vi "Main Reversi.vi"(6 "Highlight Possible Moves?":bool, 8 "error in (no error)":errorcluster, 9 "Wait per Turn (ms)":u32(slide) scale=0.0..1000.0, 10 "Games Per Match":u32=1 min=1 max=1000, 11 "Game Mode":T1(ring)) -> (0 "error out":errorcluster)   [LabVIEW 2020, in "Reversi.lvlib" / "Reversi.lvclass"]
uses:
  Reversi.lvclass
  Space Ring.ctl
  Reversi.lvclass/Reversi.ctl
  <vilib>/Utility/miscctls.llb/LVMapReplaceAction.ctl
  Player/Player.lvclass
panel:
  in  "Close":bool
  out "Win Count":i32(listbox)
  out "Running Stats":i32(listbox)
  out "Current Turn":T2
  in  "Stop":bool
  out "Board":T2[][](array[typedef])
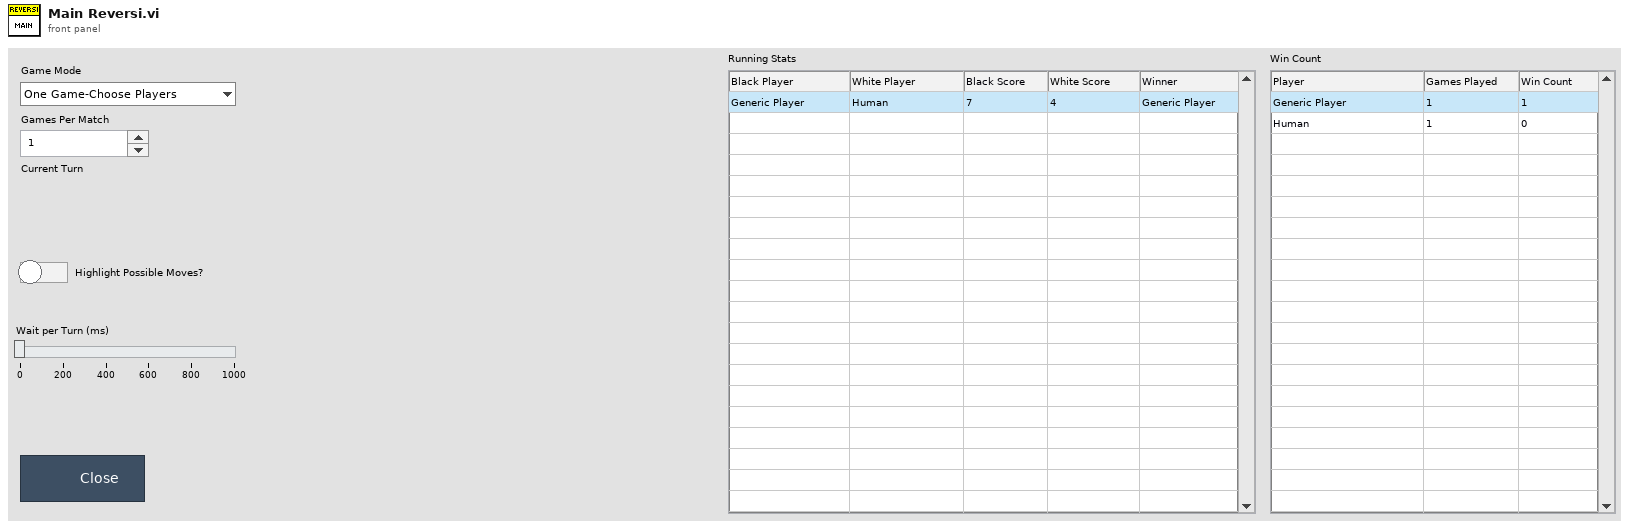
[diagram p1: front panel]
types:
  T1 = enum16{"One Game-Choose Players", "Challenge Matches (All Players)"}
  T2 = typedef "Reversi.lvlib/Reversi.lvclass/Space Ring.ctl" = u16
  T3 = cluster{"Black":refnum<class "Player.lvclass">, "White":refnum<class "Player.lvclass">}
  T4 = cluster{"Black":refnum<class "Player.lvclass">, "White":refnum<class "Player.lvclass">}[]
  T5 = cluster{"Player out":refnum<class "Player.lvclass">, "Player out":refnum<class "Player.lvclass">}
  T6 = typedef "LVMapReplaceAction.ctl" = enum32{"Modify Entry only if found", "Add or Modify Entry", "Delete Entry"}
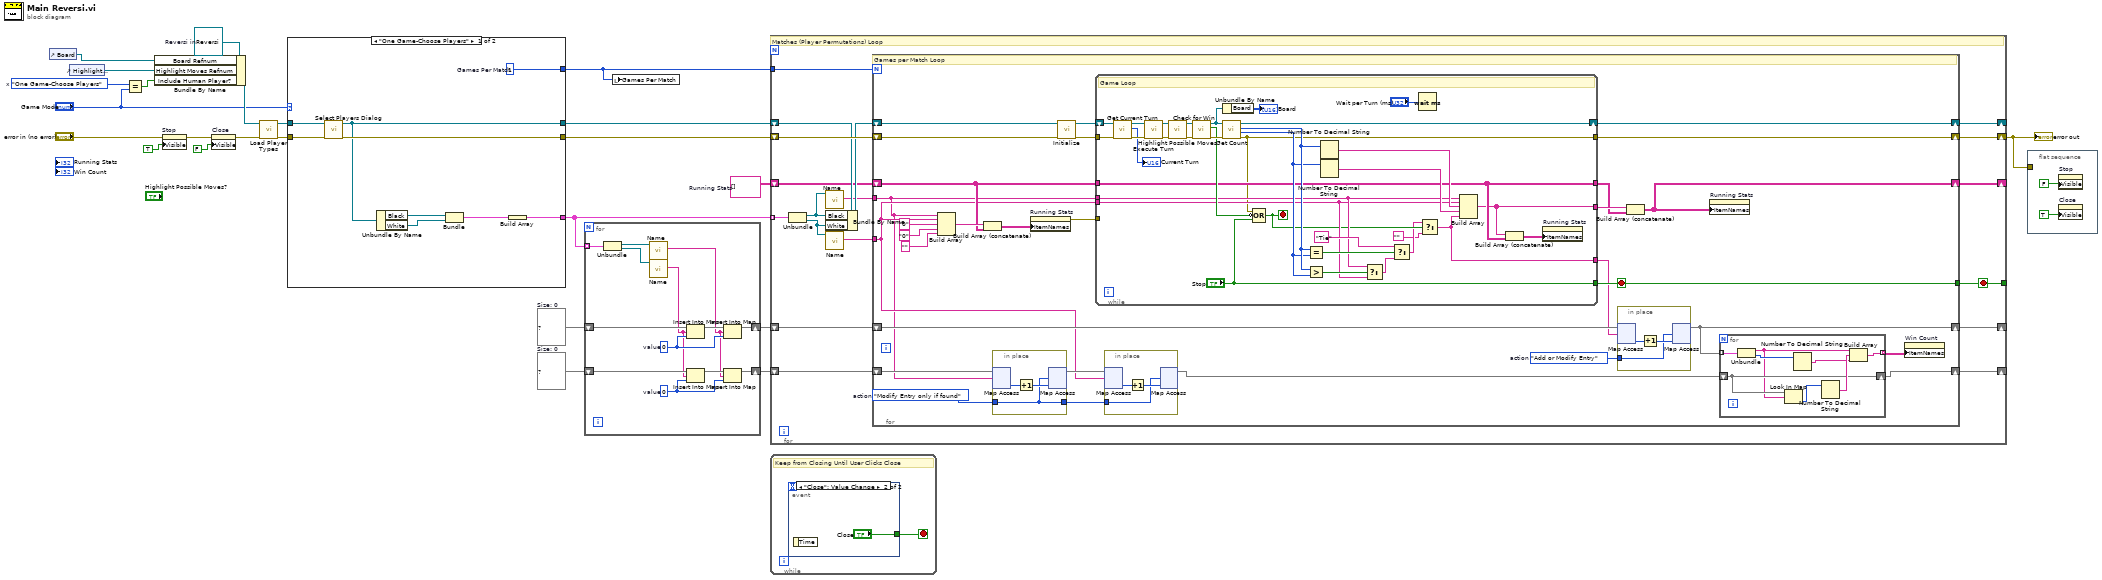
[diagram p0: block diagram]
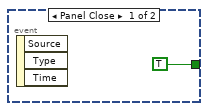
[diagram p2: hidden frame]
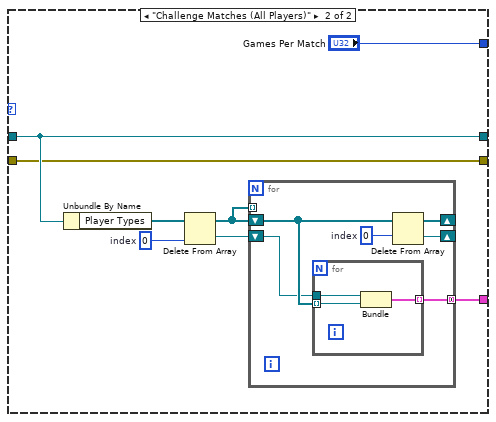
[diagram p3: hidden frame]
diagram:
  w24 = refnum<class "Reversi.lvclass"> refnum  # Reversi in
  w11 = T1."One Game-Choose Players"  # x
  w14 = map{string, i32} {}  # Size: 0
  w17 = map{string, i32} {}  # Size: 0
  w18 = string[][] []  # Running Stats
  n1 = control-ref of="Board"() -> (w6:refnum<vi>)
  n2 = control-ref of="Highlight Possible Moves?"() -> (w5:refnum<vi>)
  n3 = Equal?(x=w11, y="Game Mode") -> (x = y?=w10:bool)
  n4 = Bundle By Name(cluster=w24, "Board Refnum"=w6, "Highlight Moves Refnum"=w5, "Include Human Player?"=w10) -> (w23:refnum<class "Reversi.lvclass">)
  n5 = property on="Stop" class="Bool"(error in="error in (no error)", "Visible"=TRUE) -> (error out=w3:errorcluster)  [unwired: 1 in, 1 out]
  n6 = property on="Close" class="Bool"(error in=w3, "Visible"=FALSE) -> (error out=w4:errorcluster)  [unwired: 1 in, 1 out]
  n7 = call "Load Player Types.vi"("error in"=w4, "Reversi in"=w23) -> ("error out"=w21:errorcluster, "Reversi out"=w22:refnum<class "Reversi.lvclass">)  [unwired: 8 in]
  n8 = case shown="\"One Game-Choose Players\"" "Game Mode" {
    tunnel: [w26 w41] -> w16
    tunnel: w22 -> [w33 w36]
    tunnel: w21 -> [w32 w35]
    tunnel: [w30 w36] -> w20
    tunnel: [w31 w35] -> w19
    tunnel: [w25 "Games Per Match"] -> w9
    frame "One Game-Choose Players" {
      w25 = u32 1  # Games Per Match
      n9 = call "Select Players Dialog.vi"("error in (no error)"=w32, "Reversi in"=w33) -> ("error out"=w31:errorcluster, "Reversi out"=w30:refnum<class "Reversi.lvclass">)  [unwired: 8 in]
      n10 = Unbundle By Name(w30) -> ("Black"=w29:refnum<class "Player.lvclass">, "White"=w28:refnum<class "Player.lvclass">)
      n11 = Bundle("Black"=w29, "White"=w28) -> (w27:T3)  [unwired: 1 in]
      n12 = Build Array(w27) -> (w26:T4)
    }
    frame "Challenge Matches (All Players)" {
      w39 = 0  # index
      n13 = Unbundle By Name(w36) -> ("Player Types"=w40:refnum<class "Player.lvclass">[])
      n14 = Delete From Array(array=w40, index=w39) -> (deleted portion=w38:refnum<class "Player.lvclass">, array with subset deleted=w37:refnum<class "Player.lvclass">[])  [unwired: 1 in]
      n15 = for {
        shift-right: [w45] -> _
        shift-left: w37 -> [w46]
        tunnel: [w47] -> w41 mode=concatenating
        shift-right: [w42] -> _
        shift-left: w38 -> [w44]
        tunnel: w37 -> [_] mode=indexing
        w43 = 0  # index
        n16 = for {
          tunnel: w44 -> [w50]
          tunnel: w46 -> [w49] mode=indexing
          tunnel: [w48] -> w47 mode=indexing
          n17 = Bundle("Player out"=w50, "Player out"=w49) -> (w48:T5)  [unwired: 1 in]
        }
        n18 = Delete From Array(array=w46, index=w43) -> (deleted portion=w42:refnum<class "Player.lvclass">, array with subset deleted=w45:refnum<class "Player.lvclass">[])  [unwired: 1 in]
      }
    }
  }
  n19 = for {
    tunnel: w16 -> [w63] mode=indexing
    shift-right: [w57] -> w15
    shift-left: w17 -> [w60]
    shift-right: [w53] -> w13
    shift-left: w14 -> [w54]
    w56 = 0  # value
    w58 = 0  # value
    n20 = Unbundle(w63) -> ("Player out"=w62:refnum<class "Player.lvclass">, "Player out"=w61:refnum<class "Player.lvclass">)
    n21 = call-dynamic "Name.vi"("Player in"=w62) -> ("Name"=w52:string)  [unwired: 8 in, 2 out]
    n22 = call-dynamic "Name.vi"("Player in"=w61) -> ("Name"=w51:string)  [unwired: 8 in, 2 out]
    n23 = Insert Into Map(map in=w60, key=w51, value=w58) -> (map out=w59:map{string, i32})  [unwired: 2 out]
    n24 = Insert Into Map(map in=w54, key=w51, value=w56) -> (map out=w55:map{string, i32})  [unwired: 2 out]
    n25 = Insert Into Map(map in=w59, key=w52, value=w58) -> (map out=w57:map{string, i32})  [unwired: 2 out]
    n26 = Insert Into Map(map in=w55, key=w52, value=w56) -> (map out=w53:map{string, i32})  [unwired: 2 out]
  }
  n27 = local write "Games Per Match"(w9) -> ()
  n28 = for {
    shift-right: [w81] -> w1
    shift-left: w19 -> [w79]
    shift-right: [w80] -> _
    shift-left: w20 -> [w76]
    tunnel: w16 -> [w77] mode=indexing
    tunnel: w9 -> [w78]
    shift-right: [w69] -> _
    shift-left: w18 -> [w70]
    shift-right: [w67] -> _
    shift-left: w15 -> [w68]
    shift-right: [w65] -> _
    shift-left: w13 -> [w66]
    tunnel: [w64] -> _
    stop <- w64 stop-if-true
    # "Matches (Player Permutations) Loop"
    n29 = Unbundle(w77) -> ("Player out"=w74:refnum<class "Player.lvclass">, "Player out"=w73:refnum<class "Player.lvclass">)
    n30 = call-dynamic "Name.vi"("Player in"=w74) -> ("Name"=w72:string)  [unwired: 8 in, 2 out]
    n31 = Bundle By Name(cluster=w76, "Black"=w74, "White"=w73) -> (w75:refnum<class "Reversi.lvclass">)
    n32 = call-dynamic "Name.vi"("Player in"=w73) -> ("Name"=w71:string)  [unwired: 8 in, 2 out]
    n33 = for {
      N: w78 -> [_]
      tunnel: [w105] -> w64
      shift-right: [w110] -> w80
      shift-left: w75 -> [w109]
      shift-right: [w111] -> w81
      shift-left: w79 -> [w107]
      tunnel: w72 -> [w82]
      tunnel: w71 -> [w85]
      shift-right: [w96] -> w69
      shift-left: w70 -> [w100]
      shift-right: [w91] -> w67
      shift-left: w68 -> [w94]
      shift-right: [w83] -> w65
      shift-left: w66 -> [w89]
      stop <- w105 stop-if-true
      w88 = LVMapReplaceAction."Modify Entry only if found"  # action
      w92 = LVMapReplaceAction."Add or Modify Entry"  # action
      # "Games per Match Loop"
      n34 = Build Array(w82, w85, "0", "0", "") -> (w101:string[])
      n35 = Build Array (concatenate)(w101, w100) -> (w99:string[][])
      n36 = in-place {
        in-place-border: w88 -> [w115]
        in-place-border: [w115] -> w86
        n37 = in-place-map #1(w89, w82) -> (w117:i32)  [unwired: 1 in, 1 out]
        n38 = Increment(x=w117) -> (x+1=w116:i32)
        n39 = in-place-map #1(w116, w115) -> (w87:map{string, i32})  [unwired: 2 out]
      }
      n40 = property on="Running Stats" class="MCListbox (strict)"("ItemNames"=w99) -> (error out=w98:errorcluster)  [unwired: 2 in, 1 out]
      n41 = call "Initialize.vi"("error in"=w107, "Reversi in"=w109) -> ("error out"=w106:errorcluster, "Reversi out"=w108:refnum<class "Reversi.lvclass">)  [unwired: 8 in]
      n42 = while {
        shift-right: [w146] -> w110
        shift-left: w108 -> [w151]
        tunnel: w106 -> [w150]
        tunnel: [w118] -> w111
        tunnel: ["Stop"] -> w105
        tunnel: w100 -> [w131]
        tunnel: w98 -> [_]
        tunnel: [w131] -> w95
        tunnel: w82 -> [w134]
        tunnel: w85 -> [w133]
        tunnel: [w129] -> w97
        tunnel: [w125] -> w93
        stop <- w128 stop-if-true
        # "Game Loop"
        n43 = call "Get Current Turn.vi"("error in (no error)"=w150, "Reversi in"=w151) -> ("error out"=w148:errorcluster, "Current Turn"=→"Current Turn":T2, "Reversi out"=w149:refnum<class "Reversi.lvclass">)  [unwired: 7 in]
        n44 = call "Execute Turn.vi"("error in"=w148, "Reversi in"=w149) -> ("error out"=w120:errorcluster, "Reversi out"=w123:refnum<class "Reversi.lvclass">)  [unwired: 8 in]
        n45 = call "Highlight Possible Moves.vi"("error in (no error)"=w120, "Reversi in"=w123) -> ("error out"=w121:errorcluster, "Reversi out"=w122:refnum<class "Reversi.lvclass">)  [unwired: 8 in]
        n46 = call "Check for Win.vi"("error in (no error)"=w121, "Reversi in"=w122) -> ("error out"=w147:errorcluster, "Any Moves Left?"=w143:bool, "Reversi out"=w145:refnum<class "Reversi.lvclass">)  [unwired: 7 in]
        n47 = Unbundle By Name(w145) -> ("Board"=→"Board":T2[][])
        n48 = call "Get Count.vi"("error in (no error)"=w147, "Reversi in"=w145) -> ("error out"=w118:errorcluster, "Count of White"=w136:i16, "Count of Black"=w137:i16, "Reversi out"=w146:refnum<class "Reversi.lvclass">)  [unwired: 6 in]
        n49 = Compound Arithmetic op=OR(w118, invert w143, "Stop") -> (w128:bool)
        n50 = Equal?(x=w137, y=w136) -> (x = y?=w139:bool)
        n51 = Greater?(x=w137, y=w136) -> (0:w135:bool)
        n52 = Number To Decimal String(number=w137) -> (decimal integer string=w141:string)  [unwired: 1 in]
        n53 = Number To Decimal String(number=w136) -> (decimal integer string=w140:string)  [unwired: 1 in]
        n54 = Select(t=w134, s=w135, f=w133) -> (s? t:f=w132:string)
        n55 = Select(t="Tie", s=w139, f=w132) -> (s? t:f=w127:string)
        n56 = Wait (ms)(milliseconds to wait="Wait per Turn (ms)") -> ()  [unwired: 1 out]
        n57 = Select(t=w127, s=w128, f="") -> (s? t:f=w125:string)
        n58 = Build Array(w134, w133, w141, w140, w125) -> (w129:string[])
        n59 = Build Array (concatenate)(w129, w131) -> (w130:string[][])
        n60 = property on="Running Stats" class="MCListbox (strict)"("ItemNames"=w130) -> ()  [unwired: 2 in, 2 out]
      }
      n61 = in-place {
        in-place-border: w86 -> [w112]
        n62 = in-place-map #2(w87, w85) -> (w114:i32)  [unwired: 1 in, 1 out]
        n63 = Increment(x=w114) -> (x+1=w113:i32)
        n64 = in-place-map #2(w113, w112) -> (w84:map{string, i32})  [unwired: 2 out]
      }
      n65 = in-place {
        in-place-border: w92 -> [w160]
        n66 = in-place-map #3(w94, w93) -> (w162:i32)  [unwired: 1 in, 1 out]
        n67 = Increment(x=w162) -> (x+1=w161:i32)
        n68 = in-place-map #3(w161, w160) -> (w91:map{string, i32})  [unwired: 2 out]
      }
      n69 = Build Array (concatenate)(w97, w95) -> (w96:string[][])
      n70 = property on="Running Stats" class="MCListbox (strict)"("ItemNames"=w96) -> ()  [unwired: 2 in, 2 out]
      n71 = for {
        tunnel: w91 -> [w159] mode=indexing
        tunnel: [w157] -> w90 mode=indexing
        shift-right: [w155] -> w83
        shift-left: w84 -> [w155]
        n72 = Unbundle(w159) -> (w153:string, w158:i32)
        n73 = Look In Map(map=w155, key=w153) -> (value=w152:i32)  [unwired: 1 in, 1 out]
        n74 = Number To Decimal String(number=w158) -> (decimal integer string=w154:string)  [unwired: 1 in]
        n75 = Number To Decimal String(number=w152) -> (decimal integer string=w156:string)  [unwired: 1 in]
        n76 = Build Array(w153, w156, w154) -> (w157:string[])
      }
      n77 = property on="Win Count" class="MCListbox (strict)"("ItemNames"=w90) -> ()  [unwired: 2 in, 2 out]
    }
  }
  "error out" <- w1
  n78 = while {
    stop <- w163 stop-if-true
    # "Keep from Closing Until User Clicks Close"
    n79 = event shown="[1] \"Close\": Value Change" {
      selector: _ -> [_ _]
      dyn-events: _ -> [_ _]
      timeout: _ -> [_ _]
      tunnel: [TRUE "Close"] -> w163
      event Panel Close {
        n80 = event-data() -> ()  [unwired: 1 in, 3 out]
      }
      event "Close": Value Change {
        n81 = event-data() -> ()  [unwired: 1 in, 1 out]
      }
    }
  }
  n82 = flat-sequence {
    tunnel: w1 -> [_]
    frame #0 {
      n83 = property on="Stop" class="Bool"("Visible"=FALSE) -> ()  [unwired: 2 in, 2 out]
      n84 = property on="Close" class="Bool"("Visible"=TRUE) -> ()  [unwired: 2 in, 2 out]
    }
  }
